vi "RSZVB Set Power Calibration Method Source.vi"(8 "error in (no error)":errorcluster {"code" format="%.0x"}, 9 "Method Source (Reference Receiver After Number of Readings)":i32(ring)=1 items=["Power Meter Only", "Reference Receiver After Number of Readings", "Referene Receiver Only"], 11 "VISA resource name":refnum<visa-resource-name>) -> (0 "error out":errorcluster {"code" format="%.0x"}, 3 "VISA resource name out":refnum<visa-resource-name>)   [LabVIEW 2011]
doc: "This VI selects the source power calibration method. \n\nRemote-control command(s):\nSOURce<Ch>:POWer<Pt>:CORRection:COLLect:METHod"
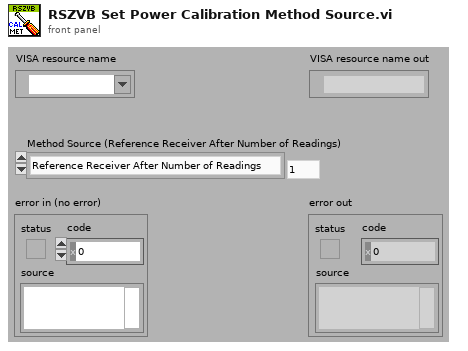
[diagram p1: front panel]
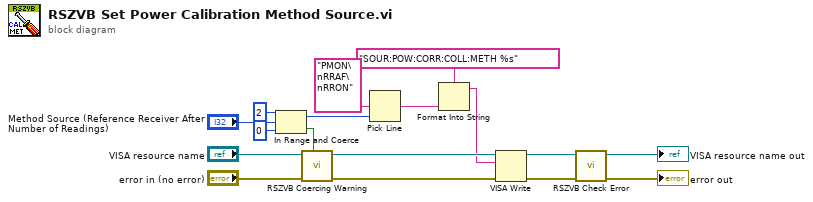
[diagram p0: block diagram]
diagram:
  n1 = In Range and Coerce(upper limit=2, x="Method Source (Reference Receiver After Number of Readings)", lower limit=0) -> (coerced(x)=w5:i32, In Range?=w8:bool)
  n2 = call "RSZVB Coercing Warning.vi"("In Range?"=w8, "error in (no error)"="error in (no error)", "VISA session"="VISA resource name") -> ("error out"=w15:errorcluster, "dup VISA session"=w14:refnum<visa-resource-name>)  [unwired: 7 in]
  n3 = Pick Line(multi-line string="PMON\nRRAF\nRRON", line index=w5) -> (output string=w1:string)  [unwired: 1 in]
  n4 = Format Into String(format string="SOUR:POW:CORR:COLL:METH %s", w1) -> (resulting string=w3:string)  [unwired: 2 in, 1 out]
  n5 = VISA Write(VISA resource name=w14, write buffer=w3, error in (no error)=w15) -> (VISA resource name out=w13:refnum<visa-resource-name>, error out=w12:errorcluster)  [unwired: 1 out]
  n6 = call "RSZVB Check Error.vi"("error in (no error)"=w12, "VISA session"=w13) -> ("error out"=→"error out":errorcluster, "dup VISA session"=→"VISA resource name out":refnum<visa-resource-name>)  [unwired: 8 in]
